vi "segementData.vi"(8 "error in (no error)":errorcluster, 9 "samplesPerChunkPerChannel":i32, 10 "segmentedData":T1(array[cluster]), 11 "SoundDeviceData in":refnum<class "SoundDeviceData.lvclass">) -> (0 "error out":errorcluster, 2 "segementData":T1(array[cluster]), 3 "SoundDeviceData out":refnum<class "SoundDeviceData.lvclass">)   [LabVIEW 2011, in "DataMappers.lvlib" / "SoundDeviceData.lvclass"]
uses:
  SoundDeviceData.lvclass
  DatabaseHelpers/Database Objects/Channel/Channel.lvclass
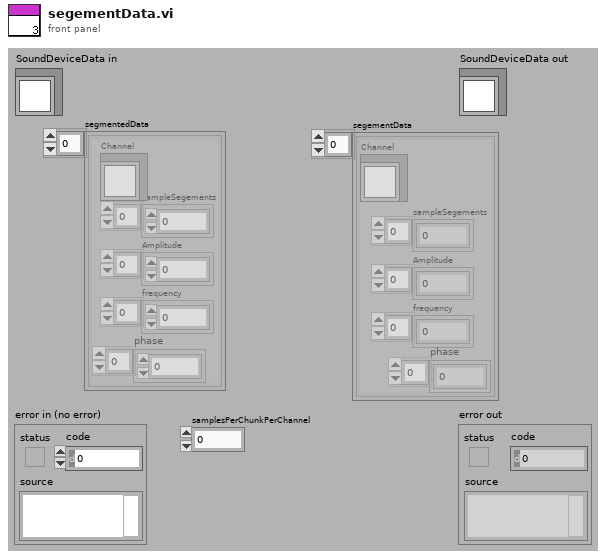
[diagram p1: front panel]
types:
  T1 = cluster{"Channel":refnum<class "Channel.lvclass">, "sampleSegements":dbl[], "Amplitude":dbl[], "frequency":dbl[], "phase":dbl[]}[]
  T2 = cluster{"Channel":refnum<class "Channel.lvclass">, "sampleSegements":dbl[], "Amplitude":dbl[], "frequency":dbl[], "phase":dbl[]}
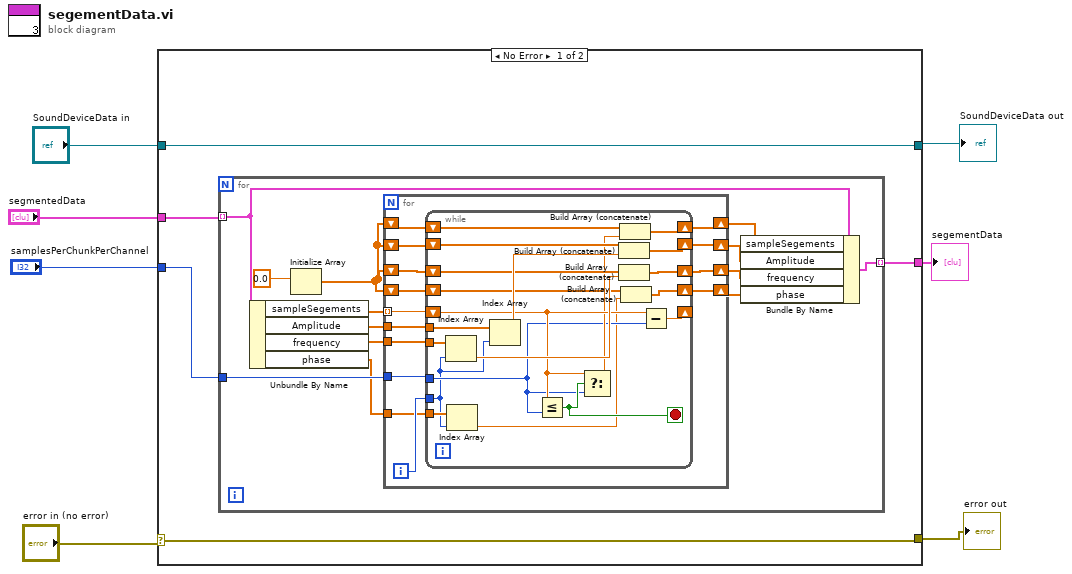
[diagram p0: block diagram]
diagram:
  n1 = case shown="No Error" "error in (no error)" {
    selector: "error in (no error)" -> [w10 w61]
    tunnel: [w10 w61] -> w6
    tunnel: [w9 w60] -> w4
    tunnel: "SoundDeviceData in" -> [w9 w60]
    tunnel: "segmentedData" -> [w12 _]
    tunnel: "samplesPerChunkPerChannel" -> [w11 _]
    tunnel: [w8 _] -> w1
    frame No Error {
      n2 = for {
        tunnel: w12 -> [w20] mode=indexing
        tunnel: w11 -> [w25]
        tunnel: [w16] -> w8 mode=indexing
        n3 = Unbundle By Name(w20) -> ("sampleSegements"=w24:dbl[], "Amplitude"=w23:dbl[], "frequency"=w22:dbl[], "phase"=w14:dbl[])
        n4 = Initialize Array(0.0) -> (w15:dbl[])  [unwired: 1 in]
        n5 = for {
          tunnel: w25 -> [w38]
          tunnel: w24 -> [w39] mode=indexing
          tunnel: w23 -> [w37]
          tunnel: w22 -> [w36]
          shift-right: [w32] -> w19
          shift-left: w15 -> [w33]
          shift-right: [w30] -> w18
          shift-left: w15 -> [w31]
          shift-right: [w29] -> w17
          shift-left: w15 -> [w34]
          shift-right: [w26] -> w13
          shift-left: w15 -> [w28]
          tunnel: w14 -> [w27]
          i -> [w35]
          n6 = while {
            tunnel: w38 -> [w45]
            tunnel: w37 -> [w57]
            tunnel: w36 -> [w58]
            shift-right: [w59] -> _
            shift-left: w39 -> [w47]
            tunnel: w35 -> [w41]
            shift-right: [w55] -> w32
            shift-left: w33 -> [w56]
            shift-right: [w53] -> w30
            shift-left: w31 -> [w54]
            shift-right: [w50] -> w29
            shift-left: w34 -> [w51]
            shift-right: [w43] -> w26
            shift-left: w28 -> [w44]
            tunnel: w27 -> [w42]
            stop <- w48 stop-if-true
            n7 = Index Array(array=w58, index=w41) -> (element=w49:dbl)
            n8 = Index Array(array=w42, index=w41) -> (element=w40:dbl)
            n9 = Index Array(array=w57, index=w41) -> (element=w52:dbl)
            n10 = Less Or Equal?(x=w47, y=w45) -> (x <= y?=w48:bool)
            n11 = Select(t=w47, s=w48, f=w45) -> (s? t:f=w46:dbl)
            n12 = Build Array (concatenate)(w54, w52) -> (w53:dbl[])
            n13 = Build Array (concatenate)(w51, w49) -> (w50:dbl[])
            n14 = Build Array (concatenate)(w56, w46) -> (w55:dbl[])
            n15 = Build Array (concatenate)(w44, w40) -> (w43:dbl[])
            n16 = Subtract(x=w47, y=w45) -> (x-y=w59:dbl)
          }
        }
        n17 = Bundle By Name(cluster=w20, "sampleSegements"=w19, "Amplitude"=w18, "frequency"=w17, "phase"=w13) -> (w16:T2)
      }
    }
    frame Error {
    }
  }
  "error out" <- w6
  "SoundDeviceData out" <- w4
  "segementData" <- w1
